vi "Construct Custom Glyph Definitions Type.vi"() -> ()   [LabVIEW 2017]
uses:
  <vilib>/gpm_packages/@cs/file-explorer-extension/Source/File Explorer/File Explorer/Custom Glyph Definition.ctl
  <vilib>/picture/picture.llb/imagedata.ctl
  <vilib>/gpm_packages/@cs/file-explorer-extension/Source/File Explorer/File Explorer/File Explorer.lvclass
panel:
  out "Custom Glyph Definitions":T1[](array[typedef])
  in  "Extension":string[](array[string])=["proc", "tmp", "set"]
  in  "PNG Path":path[](array[path])=[path "C:/Users/jonmc/Documents/Git/Test Executive Builder/Resource/Graphics/Process - Color.png", path "C:/Users/jonmc/Documents/Git/Test Executive Builder/Resource/Graphics/Temporary Process - Color.png", path "C:/Users/jonmc/Documents/Git/Test Executive Builder/Resource/Graphics/Settings - Color.png"]
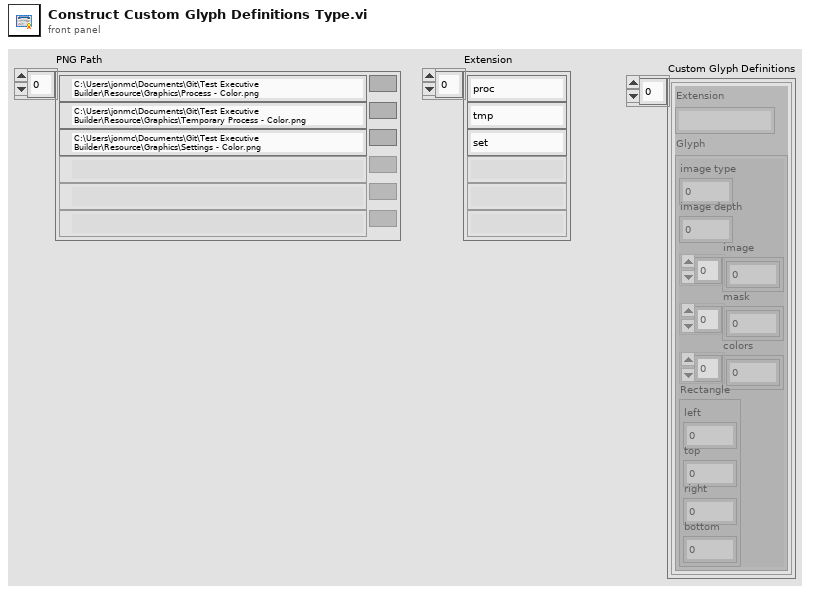
[diagram p1: front panel]
types:
  T1 = typedef "File Explorer.lvlib/File Explorer.lvclass/Custom Glyph Definition.ctl" = cluster{"Extension":string, "Glyph":T2}
  T2 = typedef "imagedata.ctl" = cluster{"image type":i32, "image depth":i32, "image":u8[], "mask":u8[], "colors":u32[], "Rectangle":cluster{"left":i16, "top":i16, "right":i16, "bottom":i16}}
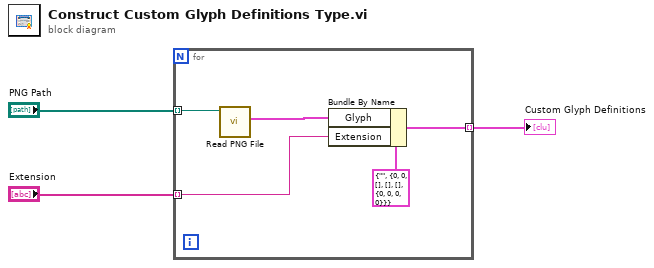
[diagram p0: block diagram]
diagram:
  n1 = for {
    tunnel: "PNG Path" -> [w8] mode=indexing
    tunnel: "Extension" -> [w5] mode=indexing
    tunnel: [w4] -> w1 mode=indexing
    n2 = call <vilib>:"Read PNG File.vi"("path to PNG file"=w8) -> ("image data"=w6:T2)  [unwired: 8 in, 2 out]
    n3 = Bundle By Name(cluster=T1 {"Extension"="", "Glyph"={"image type"=0, "image depth"=0, "image"=[], "mask"=[], "colors"=[], "Rectangle"={"left"=0, "top"=0, "right"=0, "bottom"=0}}} ("Custom Glyph Definition"), "Glyph"=w6, "Extension"=w5) -> (w4:T1)
  }
  "Custom Glyph Definitions" <- w1
